vi "Write Class Type.vi"(8 "error in (no error)":errorcluster, 10 "PDE class type":T1 items=["PDE"=0, "PDE_2ndOrder_ConstPara"=100, "PDE_Helmholtz_2D"=112, "PDE_Heat_1D"=121, "PDE_Heat_2D"=122, "PDE_Wave_1D"=131, "PDE_Wave_2D"=132], 11 "PDE.lvclass in":refnum<class "NI_PDE.lvclass">) -> (0 "error out":errorcluster, 3 "PDE.lvclass out":refnum<class "NI_PDE.lvclass">)   [LabVIEW 2020, in "NI_PDE.lvlib" / "NI_PDE.lvclass"]
uses:
  <vilib>/gmath/pde.llb/PDEClass/NI_PDE.lvclass
  <vilib>/gmath/pde.llb/PDEClass/Class Type.ctl
  <vilib>/gmath/pde.llb/PDEClass/NI_PDE.lvclass/NI_PDE.ctl
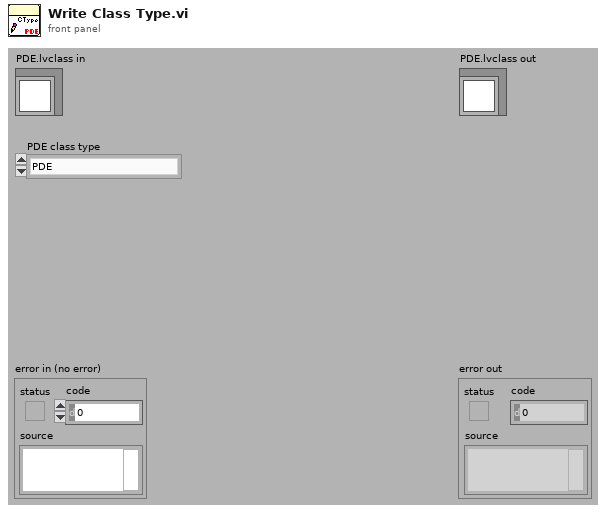
[diagram p1: front panel]
types:
  T1 = typedef "NI_PDE.lvlib/NI_PDE.lvclass/Class Type.ctl" = i32
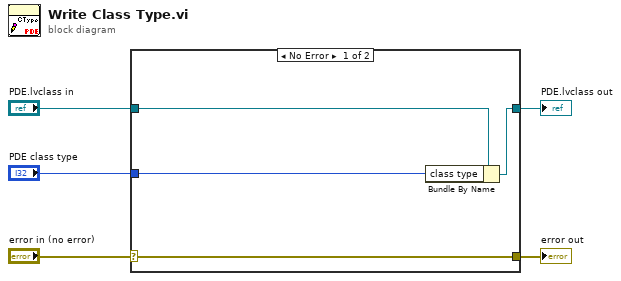
[diagram p0: block diagram]
diagram:
  n1 = case shown="No Error" "error in (no error)" {
    selector: "error in (no error)" -> [w9 w10]
    tunnel: [w9 w10] -> w4
    tunnel: [w7 w11] -> w2
    tunnel: "PDE.lvclass in" -> [w8 w11]
    tunnel: "PDE class type" -> [w6 _]
    frame No Error {
      n2 = Bundle By Name(cluster=w8, "class type"=w6) -> (w7:refnum<class "NI_PDE.lvclass">)
    }
    frame Error {
    }
  }
  "error out" <- w4
  "PDE.lvclass out" <- w2
